vi "sg Set Frequency Amplitude.vi"(8 "error in (no error)":errorcluster, 9 "amplitude":dbl, 10 "frequency":dbl, 11 "device":i32) -> (0 "error out":errorcluster, 3 "function return":u32(ring))   [LabVIEW 2014, in "VSG25A.lvlib"]
doc: "SG_API sgStatus sgSetFrequencyAmplitude(int device, double frequency, double amplitude);"
uses:
  VSG25A.lvlib
  sg_api.dll
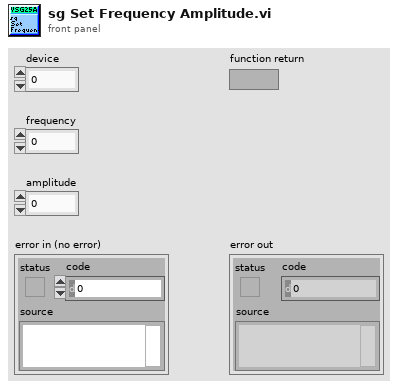
[diagram p1: front panel]
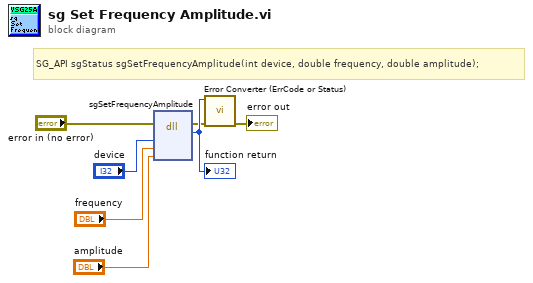
[diagram p0: block diagram]
diagram:
  # "SG_API sgStatus sgSetFrequencyAmplitude(int device, double frequency, double amplitude);"
  n1 = dll-call lib="C:/Users/M_LAPTOP/Desktop/Labview/practice/VSG25A/sg_lib/sg_api.*" fn="sgSetFrequencyAmplitude"(error in="error in (no error)", "device"="device", "frequency"="frequency", "amplitude"="amplitude") -> (error out=w2:errorcluster, w7:u32)  [unwired: 5 in, 1 out]
  "function return" <- w7
  n2 = call "Error Converter (ErrCode or Status).vi"("error in (no error)"=w2, "error code"=w7) -> ("error out"=→"error out":errorcluster)  [unwired: 9 in]
